vi "LightBoolArray.vi"(9 "BOOL Array Input in":bool[](array[boolean]), 10 "Boolean 2":bool, 11 "Boolean":bool) -> (3 "BOOL Array Input out":bool[](array[boolean]))   [LabVIEW 2015]
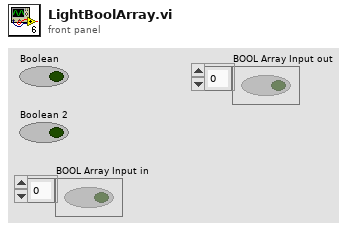
[diagram p1: front panel]
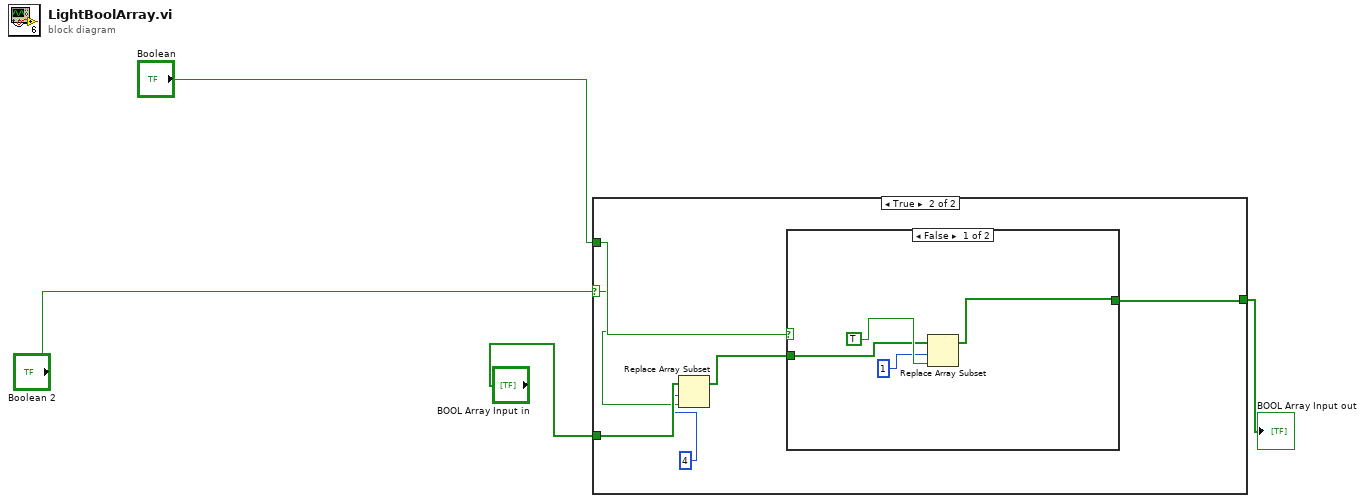
[diagram p0: block diagram]
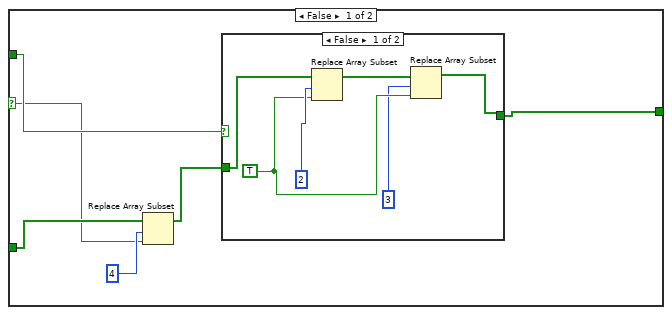
[diagram p2: hidden frame]
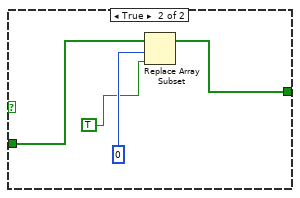
[diagram p3: hidden frame]
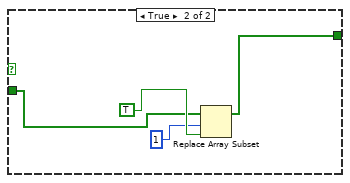
[diagram p4: hidden frame]
diagram:
  n1 = case shown="True" "Boolean 2" {
    selector: "Boolean 2" -> [w6 w22]
    tunnel: "Boolean" -> [w10 w26]
    tunnel: [w9 w25] -> w4
    tunnel: "BOOL Array Input in" -> [w8 w24]
    frame False {
      n2 = Replace Array Subset(array=w8, new element=w6, index=4) -> (w5:bool[])
      n3 = case shown="False" w10 {
        tunnel: [w11 w17] -> w9
        tunnel: w5 -> [w16 w20]
        frame False {
          w13 = TRUE
          n4 = Replace Array Subset(array=w16, new element=w13, index=2) -> (w15:bool[])
          n5 = Replace Array Subset(array=w15, new element=w13, index=3) -> (w11:bool[])
        }
        frame True {
          n6 = Replace Array Subset(array=w20, new element=TRUE, index=0) -> (w17:bool[])
        }
      }
    }
    frame True {
      n7 = Replace Array Subset(array=w24, new element=w22, index=4) -> (w21:bool[])
      n8 = case shown="False" w26 {
        tunnel: [w27 w31] -> w25
        tunnel: w21 -> [w28 w32]
        frame False {
          n9 = Replace Array Subset(array=w28, new element=TRUE, index=1) -> (w27:bool[])
        }
        frame True {
          n10 = Replace Array Subset(array=w32, new element=TRUE, index=1) -> (w31:bool[])
        }
      }
    }
  }
  "BOOL Array Input out" <- w4
